vi "Lire Parameters.vi"(11 "Exchange en entrée":refnum<class "Exchange.lvclass">) -> (2 "Parameters":T1 {"Currency" items=["Euro", "Dollar", "Yen", "RIM", "CHF"]}, 3 "Exchange en sortie":refnum<class "Exchange.lvclass">)   [LabVIEW 2012, in "Exchange.lvclass"]
uses:
  Exchange.lvclass
  Exchange Parameters.ctl
  Exchange Type Enum.ctl
  controls/Currencies.ctl
  Exchange.lvclass/Exchange.ctl
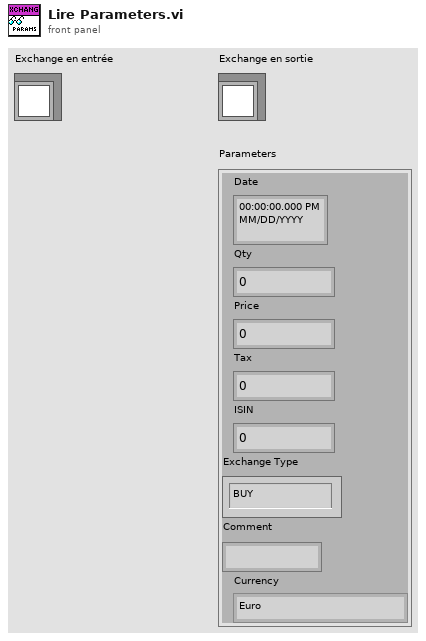
[diagram p1: front panel]
types:
  T1 = typedef "Exchange Parameters.ctl" = cluster{"Date":timestamp, "Qty":dbl, "Price":dbl, "Tax":dbl, "ISIN":dbl, "Exchange Type":T2, "Comment":string, "Currency":T3}
  T2 = typedef "Exchange.lvclass/Exchange Type Enum.ctl" = enum16{"BUY", "SELL"}
  T3 = typedef "Currencies.ctl" = u16
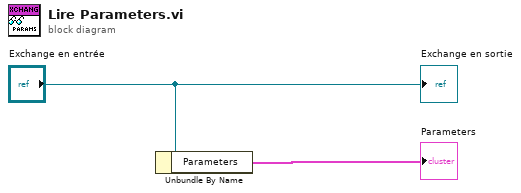
[diagram p0: block diagram]
diagram:
  n1 = Unbundle By Name("Exchange en entrée") -> ("Parameters"=→"Parameters":T1)
  "Exchange en sortie" <- "Exchange en entrée"
